vi "PH_gentec_P-Link.Action set Settings.vi"(0 "i ref in":refnum<vi>, 5 "error in":errorcluster) -> (14 "i ref out":refnum<vi>, 19 "error out":errorcluster)   [LabVIEW 2014, in "PH_gentec_P-Link.lvlib"]
doc: "This VI sets the device to the wanted settings."
uses:
  PH_gentec_P-Link.lvlib
  PH_Basics/PH_Powermeter_BaseClass/PH_Powermeter_BaseClass.State.ctl
  PH_Basics/PH_Powermeter_BaseClass/PH_Powermeter_BaseClass.lvlib
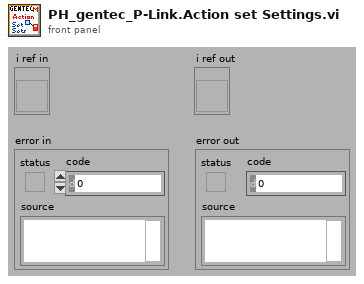
[diagram p1: front panel]
types:
  T1 = typedef "PH_Powermeter_BaseClass.lvlib/PH_Powermeter_BaseClass.State.ctl" = enum32{"off", "operating", "opened", "checked", "connected", "Sets to change", "running"}
  T2 = typedef "PH_Powermeter_BaseClass.lvlib/PH_Powermeter_BaseClass.i attribute.ctl" = cluster{"GUI References":T3, "Connection":T4, "Head Attributes":T5, "VISA resource":refnum<visa-resource-name>, "Energy":T6, "Service ID Energy":i32, "Wanted Settings":T7, "Current Settings":T7}
  T3 = typedef "PH_Powermeter_BaseClass.lvlib/PH_Powermeter_BaseClass.GUI Refs.ctl" = cluster{"Head Attributes":refnum<vi>, "Energy":refnum<vi>, "Connection":refnum<vi>, "VISA Resource":refnum<vi>, "Energy evolution":refnum<vi>, "Scaling Factor":refnum<vi>, "Range":refnum<vi>, "Wavelength":refnum<vi>, "Trigger Level":refnum<vi>, "Wanted Settings":refnum<vi>, "Current Settings":refnum<vi>}
  T4 = typedef "PH_Powermeter_BaseClass.lvlib/PH_Powermeter_BaseClass.Connection.ctl" = cluster{"failed checks":i8, "Timeout":bool, "Data read":string, "Failure":bool, "Error":bool, "State":T1}
  T5 = typedef "PH_Powermeter_BaseClass.lvlib/PH_Powermeter_BaseClass.Head Attributes.ctl" = cluster{"Instrument Type":string, "Head Version":string, "Head Name":string, "Serial Number":string, "Firmware":string, "Sensor Type":string, "MinimumRange":u32, "Maximum Range":u32, "Min Wavelength":i32, "Max Wavelength":i32}
  T6 = typedef "PH_Powermeter_BaseClass.lvlib/PH_Powermeter_BaseClass.Energy.ctl" = cluster{"current Value":dbl, "unscaled":dbl, "Scaling Factor":dbl}
  T7 = typedef "PH_Powermeter_BaseClass.lvlib/PH_gentec_BaseClass.Head Settings.ctl" = cluster{"Trigger Level":dbl, "Wavelength":u32, "Range":u32}
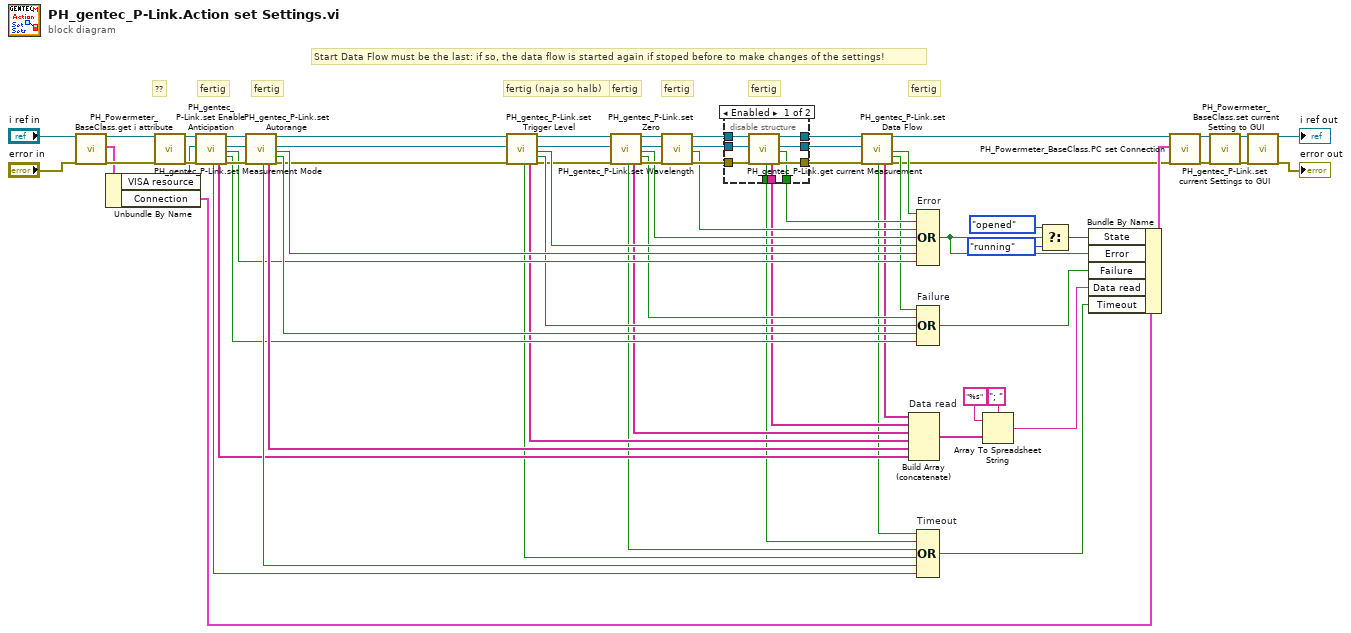
[diagram p0: block diagram]
diagram:
  # "fertig"
  # "fertig"
  # "fertig"
  # "fertig"
  # "fertig (naja so halb)"
  # "fertig"
  # "??"
  # "fertig"
  # "Start Data Flow must be the last: if so, the data flow is started again if stoped before to make changes of the settings!"
  n1 = call "PH_Powermeter_BaseClass.get i attribute.vi"("i ref in"="i ref in", "error in (no error)"="error in") -> ("i ref out"=w18:refnum<vi>, "i attribute"=w15:T2, "error out"=w16:errorcluster)  [unwired: 15 in]
  n2 = Unbundle By Name(w15) -> ("VISA resource"=w14:refnum<visa-resource-name>, "Connection"=w13:T4)
  n3 = call "PH_gentec_P-Link.set Measurement Mode.vi"("i ref in"=w18, "error in"=w16) -> ("i ref out"=w67:refnum<vi>, "error out"=w69:errorcluster)  [unwired: 16 in]
  n4 = call "PH_gentec_P-Link.set Enable Anticipation.vi"("i ref in"=w67, "VISA resource in"=w14, "error in"=w69) -> ("Timeout"=w56:bool, "Data read"=w57:string[], "i ref out"=w66:refnum<vi>, "VISA resource out"=w65:refnum<visa-resource-name>, "Error"=w54:bool, "Failure"=w55:bool, "error out"=w68:errorcluster)  [unwired: 10 in]
  n5 = call "PH_gentec_P-Link.set Autorange.vi"("i ref in"=w66, "VISA resource in"=w65, "error in"=w68) -> ("Timeout"=w64:bool, "Data read"=w59:string[], "i ref out"=w6:refnum<vi>, "VISA resource out"=w4:refnum<visa-resource-name>, "Error"=w62:bool, "Failure"=w61:bool, "error out"=w5:errorcluster)  [unwired: 10 in]
  n6 = call "PH_gentec_P-Link.set Trigger Level.vi"("i ref in"=w6, "VISA resource in"=w4, "error in"=w5) -> ("Timeout"=w50:bool, "Data read"=w51:string[], "i ref out"=w3:refnum<vi>, "VISA resource out"=w1:refnum<visa-resource-name>, "Error"=w53:bool, "Failure"=w52:bool, "error out"=w2:errorcluster)  [unwired: 10 in]
  n7 = call "PH_gentec_P-Link.set Wavelength.vi"("i ref in"=w3, "VISA resource in"=w1, "error in"=w2) -> ("Timeout"=w48:bool, "Data read"=w47:string[], "i ref out"=w42:refnum<vi>, "VISA resource out"=w43:refnum<visa-resource-name>, "Error"=w45:bool, "Failure"=w46:bool, "error out"=w49:errorcluster)  [unwired: 10 in]
  n8 = call "PH_gentec_P-Link.set Zero.vi"("i ref in"=w42, "VISA resource in"=w43, "error in"=w49) -> ("i ref out"=w39:refnum<vi>, "VISA resource out"=w38:refnum<visa-resource-name>, "Error"=w41:bool, "error out"=w44:errorcluster)  [unwired: 13 in]
  n9 = disable-structure shown="Enabled" {
    disable-tunnel: w44 -> [w79 w80]
    disable-tunnel: [w78 w80] -> w40
    disable-tunnel: w39 -> [w77 w82]
    disable-tunnel: w38 -> [w76 w81]
    disable-tunnel: [w75 _] -> w37
    disable-tunnel: [w74 _] -> w36
    disable-tunnel: [w73 _] -> w35
    disable-tunnel: [w72 w82] -> w34
    disable-tunnel: [w71 w81] -> w33
    frame Enabled {
      n10 = call "PH_gentec_P-Link.get current Measurement.vi"("i ref in"=w77, "VISA resource in"=w76, "error in"=w79) -> ("Timeout"=w75:bool, "Data read"=w74:string[], "i ref out"=w72:refnum<vi>, "VISA resource out"=w71:refnum<visa-resource-name>, "Error"=w73:bool, "error out"=w78:errorcluster)  [unwired: 11 in]
    }
    frame Disabled {
    }
  }
  n11 = call "PH_gentec_P-Link.set Data Flow.vi"("i ref in"=w34, "VISA resource in"=w33, "error in"=w40) -> ("Timeout"=w32:bool, "Data read"=w29:string[], "i ref out"=w24:refnum<vi>, "Error"=w31:bool, "Failure"=w30:bool, "error out"=w23:errorcluster)  [unwired: 10 in, 1 out]
  n12 = Build Array (concatenate) "Data read"(w29, w36, w47, w51, w59, w57) -> (w58:string[])
  n13 = Compound Arithmetic op=OR "Error"(w31, w35, w41, w45, w53, w62, w54) -> (w22:bool)
  n14 = Compound Arithmetic op=OR "Failure"(w30, w46, w52, w61, w55) -> (w60:bool)
  n15 = Compound Arithmetic op=OR "Timeout"(w32, w37, w48, w50, w64, w56) -> (w63:bool)
  n16 = Array To Spreadsheet String(delimiter (Tab)="; ", array=w58, 3:"%s" ("format string")) -> (spreadsheet string=w26:string)
  n17 = Select(t=PH_Powermeter_BaseClass.State."opened" ("State"), s=w22, f=PH_Powermeter_BaseClass.State."running") -> (s? t:f=w20:T1)
  n18 = Bundle By Name(cluster=w13, "State"=w20, "Error"=w22, "Failure"=w60, "Data read"=w26, "Timeout"=w63) -> (w25:T4)
  n19 = call "PH_Powermeter_BaseClass.PC set Connection.vi"("VI in"=w24, "Connection"=w25, "error in (no error)"=w23) -> ("VI out"=w12:refnum<vi>, "error out"=w10:errorcluster)  [unwired: 15 in]
  n20 = call "PH_gentec_P-Link.set current Settings to GUI.vi"("i ref in"=w12, "error in"=w10) -> ("i ref out"=w8:refnum<vi>, "error out"=w11:errorcluster)  [unwired: 16 in]
  n21 = call "PH_Powermeter_BaseClass.set current Setting to GUI.vi"("VI in"=w8, "error in (no error)"=w11) -> ("VI out"=→"i ref out":refnum<vi>, "error out"=→"error out":errorcluster)  [unwired: 16 in]
